vi "hp83623a Init and Update.vi"(8 "error in (no error)":errorcluster, 11 "hp83623a Settings (in)":T1={"Frequency (Hz)"=0.0, "Power (dBm)"=0.0, "Enabled"=TRUE, "initialized"=FALSE, "RF Output On/Off"=TRUE, "External Trigger?"=FALSE, "VISA Session"="GPIB0::3::INSTR", "Generator Name"="Generator"}) -> (0 "error out":errorcluster, 3 "hp83623a Settings":T1={"Frequency (Hz)"=0.0, "Power (dBm)"=0.0, "Enabled"=TRUE, "initialized"=FALSE, "RF Output On/Off"=TRUE, "External Trigger?"=FALSE, "VISA Session"="GPIB0::3::INSTR", "Generator Name"="Generator"})   [LabVIEW 2013, in "HP83623A_RF_Generator.lvclass"]
uses:
  HP83623A_RF_Generator.lvclass
  HP83623A.ctl
  Experiment/Globals.vi
panel:
  in  "Source(Internal:0)":u16(ring)=1 items=["Internal", "External", "Scalar"]
  in  "Ampiltude Mode (Fixed/single output level:2)":u16(ring)=2 items=["sweep         starting power        ending power", "sweep         center power                 span", "Fixed           single output level       (no effect)"]
  in  "Frequency Mode (CW mode: 2)":u16(ring)=2 items=["sweep           start frequency     stop frequency", "sweep         center frequency   frequency span", "CW mode    single frequency       (no effect)", "Manual        single frequency       (no effect)"]
  in  "Frequency Operation(Fixed:0)":u16(ring)=1 items=["Fixed", "CW", "Sweep", "List"]
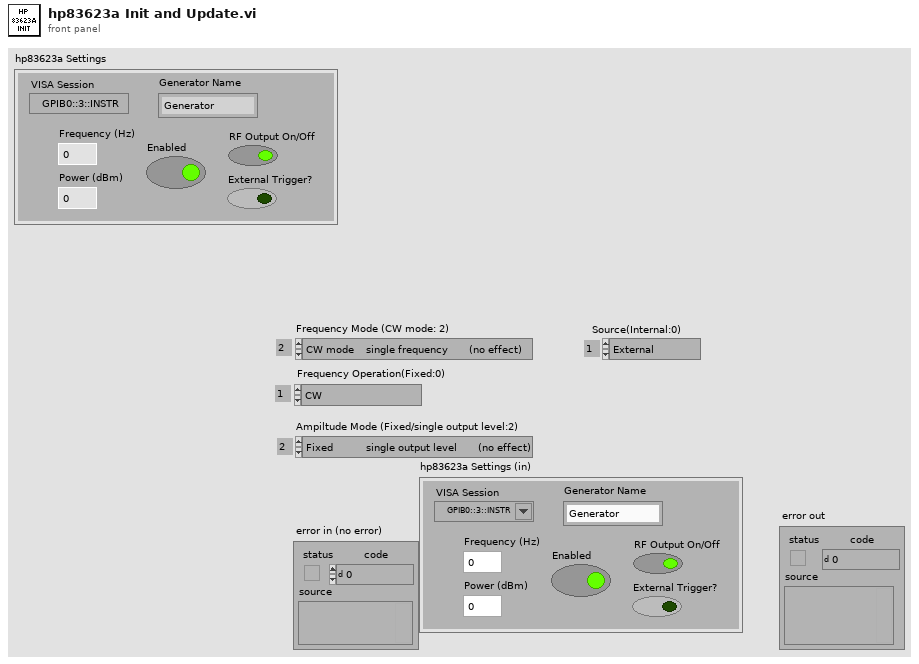
[diagram p1: front panel]
types:
  T1 = typedef "HP83623A_RF_Generator.lvclass/HP83623A.ctl" = cluster{"Frequency (Hz)":dbl, "Power (dBm)":dbl, "Enabled":bool, "initialized":bool, "RF Output On/Off":bool, "External Trigger?":bool, "VISA Session":refnum<visa-resource-name>, "Generator Name":string}
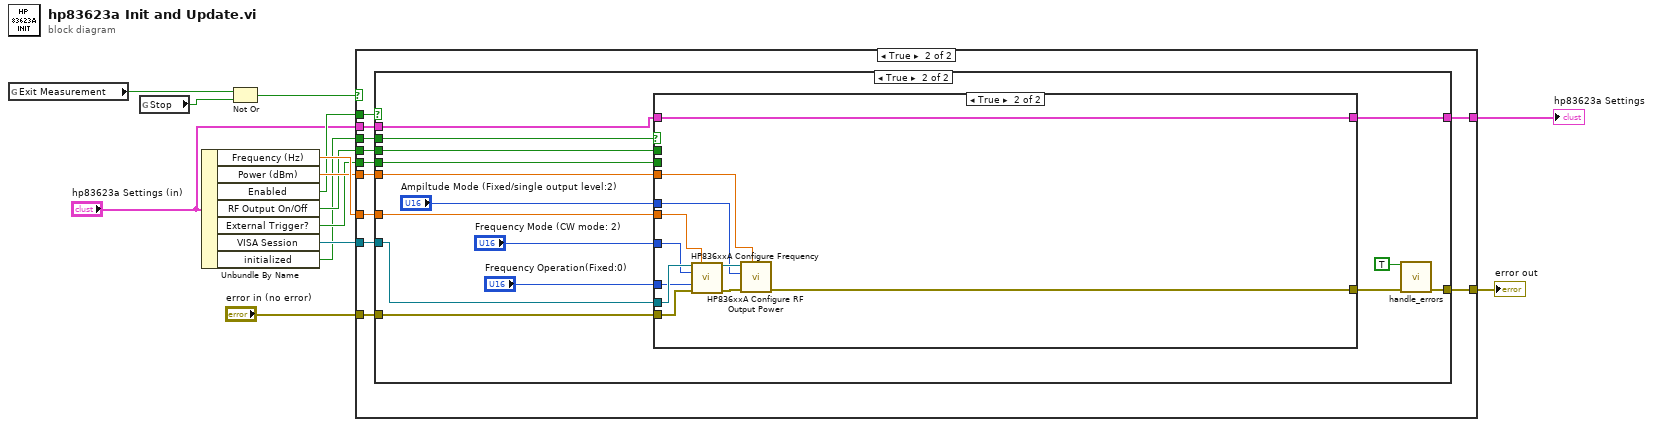
[diagram p0: block diagram]
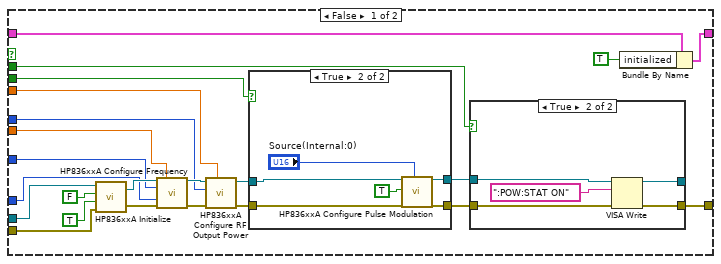
[diagram p4: hidden frame]
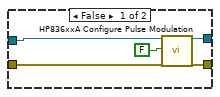
[diagram p5: hidden frame]
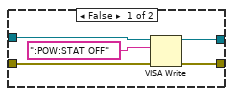
[diagram p6: hidden frame]
diagram:
  n1 = global read "Globals.vi" "Exit Measurement"() -> (w5:bool)
  n2 = global read "Globals.vi" "Stop"() -> (w4:bool)
  n3 = Unbundle By Name("hp83623a Settings (in)") -> ("Frequency (Hz)"=w13:dbl, "Power (dBm)"=w12:dbl, "Enabled"=w11:bool, "RF Output On/Off"=w10:bool, "External Trigger?"=w9:bool, "VISA Session"=w14:refnum<visa-resource-name>, "initialized"=w8:bool)
  n4 = Not Or(1:w4, 2:w5) -> (0:w2:bool)
  n5 = case shown="True" w2 {
    tunnel: w14 -> [_ w27]
    tunnel: [w15 w26] -> w1
    tunnel: w13 -> [_ w25]
    tunnel: w12 -> [_ w24]
    tunnel: w11 -> [_ w23]
    tunnel: w10 -> [_ w22]
    tunnel: w9 -> [_ w21]
    tunnel: "hp83623a Settings (in)" -> [w16 w20]
    tunnel: [w16 w19] -> w6
    tunnel: w8 -> [_ w18]
    tunnel: "error in (no error)" -> [w15 w17]
    frame False {
    }
    frame True {
      n6 = case shown="True" w23 {
        tunnel: w27 -> [_ w44]
        tunnel: w17 -> [w29 w38]
        tunnel: [w29 w30] -> w26
        tunnel: w25 -> [_ w39]
        tunnel: w24 -> [_ w37]
        tunnel: w22 -> [_ w43]
        tunnel: w21 -> [_ w42]
        tunnel: w20 -> [w28 w41]
        tunnel: [w28 w40] -> w19
        tunnel: w18 -> [_ w36]
        frame False {
        }
        frame True {
          n7 = case shown="True" w36 {
            tunnel: w44 -> [w67 w96]
            tunnel: w43 -> [w66 _]
            tunnel: w42 -> [w65 _]
            tunnel: w41 -> [w64 w97]
            tunnel: [w63 w97] -> w40
            tunnel: w39 -> [w46 w90]
            tunnel: w38 -> [w47 w91]
            tunnel: w37 -> [w45 w89]
            tunnel: [w62 w95] -> w31
            tunnel: "Ampiltude Mode (Fixed/single output level:2)" -> [w50 w94]
            tunnel: "Frequency Mode (CW mode: 2)" -> [w49 w93]
            tunnel: "Frequency Operation(Fixed:0)" -> [w48 w92]
            frame False {
              n8 = call "HP836xxA Initialize.vi"("error in (no error)"=w47, "reset"=TRUE, "ID query"=FALSE, "VISA Session"=w67) -> ("error out"=w54:errorcluster, "dup VISA session"=w61:refnum<visa-resource-name>)
              n9 = call "HP836xxA Configure Frequency.vi"("VISA session"=w61, "freq 1"=w46, "Mode (CW mode: 2)"=w49, "Operation(Fixed:0)"=w48, "error in (no error)"=w54) -> ("dup VISA session"=w59:refnum<visa-resource-name>, "error out"=w60:errorcluster)  [unwired: 9 in]
              n10 = call "HP836xxA Configure RF Output Power.vi"("power 1"=w45, "error in (no error)"=w60, "Mode (Fixed/single output level:2)"=w50, "VISA session"=w59) -> ("error out"=w57:errorcluster, "dup VISA session"=w58:refnum<visa-resource-name>)  [unwired: 6 in]
              n11 = case shown="True" w65 {
                tunnel: w58 -> [w71 w78]
                tunnel: w57 -> [w70 w77]
                tunnel: [w68 w76] -> w56
                tunnel: [w69 w75] -> w55
                frame False {
                  n12 = call "HP836xxA Configure Pulse Modulation.vi"("VISA session"=w71, "State(Off:F)"=FALSE, "error in (no error)"=w70) -> ("dup VISA session"=w68:refnum<visa-resource-name>, "error out"=w69:errorcluster)  [unwired: 15 in]
                }
                frame True {
                  n13 = call "HP836xxA Configure Pulse Modulation.vi"("VISA session"=w78, "State(Off:F)"=TRUE, "error in (no error)"=w77, "Source(Internal:0)"="Source(Internal:0)") -> ("dup VISA session"=w76:refnum<visa-resource-name>, "error out"=w75:errorcluster)  [unwired: 14 in]
                }
              }
              n14 = case shown="True" w66 {
                tunnel: w56 -> [w81 w88]
                tunnel: w55 -> [w80 w87]
                tunnel: [w79 w86] -> _
                tunnel: [w82 w85] -> w62
                frame False {
                  n15 = VISA Write(VISA resource name=w81, write buffer=":POW:STAT OFF", error in (no error)=w80) -> (VISA resource name out=w79:refnum<visa-resource-name>, error out=w82:errorcluster)  [unwired: 1 out]
                }
                frame True {
                  n16 = VISA Write(VISA resource name=w88, write buffer=":POW:STAT ON", error in (no error)=w87) -> (VISA resource name out=w86:refnum<visa-resource-name>, error out=w85:errorcluster)  [unwired: 1 out]
                }
              }
              n17 = Bundle By Name(cluster=w64, "initialized"=TRUE ("83623 initialized")) -> (w63:T1)
            }
            frame True {
              n18 = call "HP836xxA Configure Frequency.vi"("VISA session"=w96, "freq 1"=w90, "Mode (CW mode: 2)"=w93, "Operation(Fixed:0)"=w92, "error in (no error)"=w91) -> ("dup VISA session"=w98:refnum<visa-resource-name>, "error out"=w99:errorcluster)  [unwired: 9 in]
              n19 = call "HP836xxA Configure RF Output Power.vi"("power 1"=w89, "error in (no error)"=w99, "Mode (Fixed/single output level:2)"=w94, "VISA session"=w98) -> ("error out"=w95:errorcluster)  [unwired: 6 in, 1 out]
            }
          }
          n20 = call "handle_errors.vi"("Exit Operation"=TRUE, "error in (no error)"=w31) -> ("error out"=w30:errorcluster)  [unwired: 13 in]
        }
      }
    }
  }
  "error out" <- w1
  "hp83623a Settings" <- w6
